vi "RenameDNS.vi"(8 "error in (no error)":errorcluster, 10 "Targets in":T3 {"Filtered Targets"."IP Mode" items=["Static"=1, "DHCP/Link-Local"=2, "Link-Local Only"=4, "DHCP Only"=8]}, 11 "Ctl Refs in":T6) -> (0 "error out":errorcluster, 2 "Targets out":T3 {"Filtered Targets"."IP Mode" items=["Static"=1, "DHCP/Link-Local"=2, "Link-Local Only"=4, "DHCP Only"=8]}, 4 "Buttons out":T2, 5 "Execution State out":T1)   [LabVIEW 2013]
uses:
  Controls/Refs.ctl
  Controls/Button Refs.ctl
  Controls/Tab Ctl Refs.ctl
  types/TabStateType.ctl
  Controls/Indicator Refs.ctl
  Controls/Slider Refs.ctl
  Controls/Control Refs.ctl
  Controls/Targets.ctl
  Controls/Detected.ctl
  types/MAX Sys Cfg Target Information.ctl
  types/ButtonStateType.ctl
  types/ExecutionStateType.ctl
  <vilib>/nisyscfg/Save Changes (System).vi
  <vilib>/nisyscfg/Close (System).vi
  <vilib>/nisyscfg/nisyscfg.lvlib
  <resource>/objmgr/nisysapi.rc
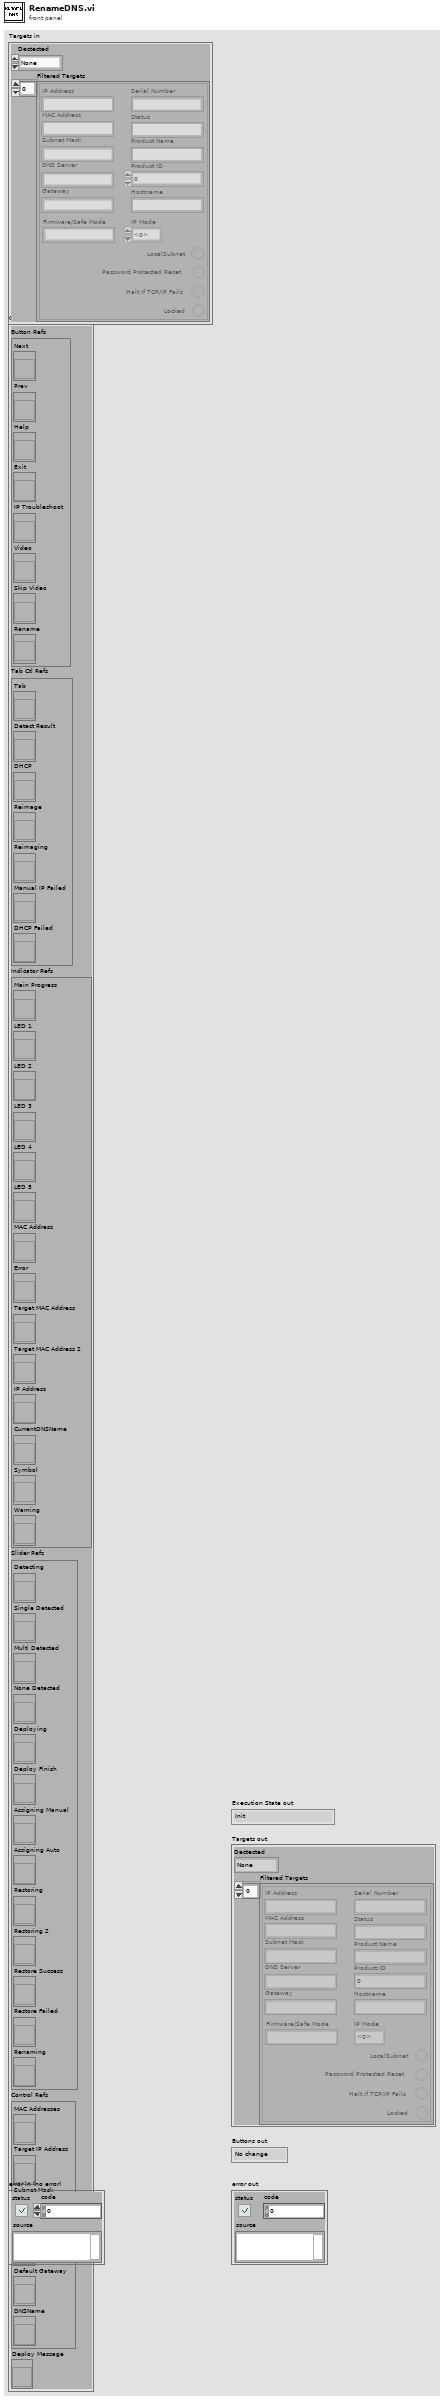
[diagram p1: front panel]
types:
  T1 = typedef "ExecutionStateType.ctl" = enum16{"Init", "Welcome", "Idle", "Detect", "Run Detection", "Detect Fail", "Detect One", "Detect Mult", "Deploy", "DHCP", "Static IP", "Run Deployment", "Connect Verify", "Exit", "Video Wait", "Success", "Troubleshoot", "Troubleshoot 2", "RenameDNS"}
  T2 = typedef "ButtonStateType.ctl" = enum16{"No change", "No Next", "No Prev", "All Disabled", "All Enabled", "Exit Only"}
  T3 = typedef "Targets.ctl" = cluster{"Dectected":T4, "Filtered Targets":T5[]}
  T4 = typedef "Detected.ctl" = enum16{"None", "Failed", "Single", "Multi"}
  T5 = typedef "MAX Sys Cfg Target Information.ctl" = cluster{"MAC Address":string, "IP Address":string, "Status":string, "Product Name":string, "Hostname":string, "Firmware/Safe Mode":string, "Subnet Mask":string, "Gateway":string, "DNS Server":string, "Serial Number":string, "Product ID":u32, "Locked ":bool, "LocalSubnet":bool, "Halt If TCP/IP Fails":bool, "Password Protected Reset":bool, "IP Mode":i32}
  T6 = typedef "Refs.ctl" = cluster{"Button Refs":T7, "Tab Ctl Refs":T8, "Indicator Refs":T9, "Slider Refs":T10, "Control Refs":T11, "Deploy Message":refnum<vi>}
  T7 = typedef "Button Refs.ctl" = cluster{"Next":refnum<vi>, "Prev":refnum<vi>, "Help":refnum<vi>, "Exit":refnum<vi>, "IP Troubleshoot":refnum<vi>, "Video":refnum<vi>, "Skip Video":refnum<vi>, "Rename":refnum<vi>}
  T8 = typedef "Tab Ctl Refs.ctl" = cluster{"Tab":refnum<vi>, "Detect Result":refnum<vi>, "DHCP":refnum<vi>, "Reimage":refnum<vi>, "Reimaging":refnum<vi>, "Manual IP Failed":refnum<vi>, "DHCP Failed":refnum<vi>}
  T9 = typedef "Indicator Refs.ctl" = cluster{"Main Progress":refnum<vi>, "LED 1":refnum<vi>, "LED 2":refnum<vi>, "LED 3":refnum<vi>, "LED 4":refnum<vi>, "LED 5":refnum<vi>, "MAC Address":refnum<vi>, "Error":refnum<vi>, "Target MAC Address":refnum<vi>, "Target MAC Address 2":refnum<vi>, "IP Address":refnum<vi>, "CurrentDNSName":refnum<vi>, "Symbol":refnum<vi>, "Warning":refnum<vi>}
  T10 = typedef "Slider Refs.ctl" = cluster{"Detecting":refnum<vi>, "Single Detected":refnum<vi>, "Multi Detected":refnum<vi>, "None Detected":refnum<vi>, "Deploying":refnum<vi>, "Deploy Finish":refnum<vi>, "Assigning Manual":refnum<vi>, "Assigning Auto":refnum<vi>, "Restoring":refnum<vi>, "Restoring 2":refnum<vi>, "Restore Success":refnum<vi>, "Restore Failed":refnum<vi>, "Renaming":refnum<vi>}
  T11 = typedef "Control Refs.ctl" = cluster{"MAC Addresses":refnum<vi>, "Target IP Address":refnum<vi>, "Subnet Mask":refnum<vi>, "DNS IP":refnum<vi>, "Default Gateway":refnum<vi>, "DNSName":refnum<vi>}
  T12 = typedef "TabStateType.ctl" = enum32{"Welcome", "Instructions", "Detect", "Run Detection", "Detect Result", "Deploy", "Run Deployment", "Connect Verify", "Success", "DHCP", "Troubleshoot", "System Restore", "Error", "Video", "Rename"}
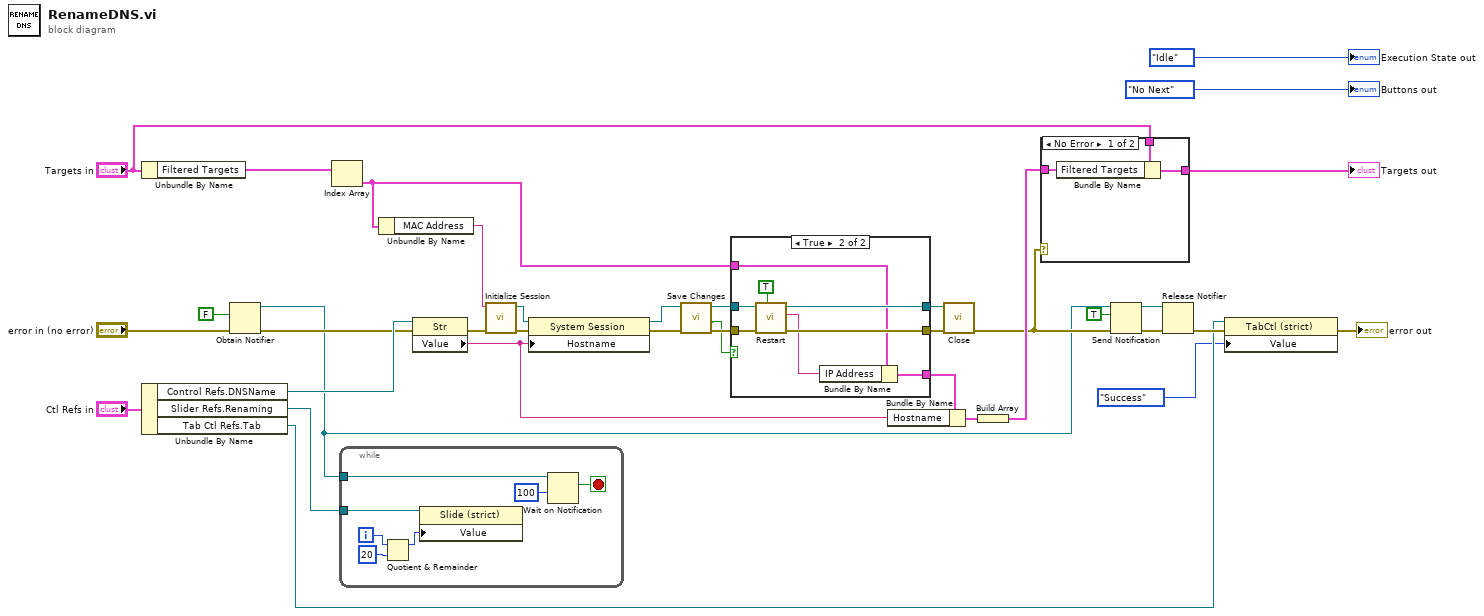
[diagram p0: block diagram]
diagram:
  n1 = Unbundle By Name("Targets in") -> ("Filtered Targets"=w36:T5[])
  n2 = Unbundle By Name("Ctl Refs in") -> ("Control Refs.DNSName"=w22:refnum<vi>, "Slider Refs.Renaming"=w11:refnum<vi>, "Tab Ctl Refs.Tab"=w2:refnum<vi>)
  n3 = Obtain Notifier(notification data type=FALSE ("wait until complete (T)"), error in (no error)="error in (no error)") -> (notifier out=w7:refnum<notifier>, error out=w10:errorcluster)  [unwired: 2 in, 1 out]
  n4 = Index Array(array=w36) -> (element=w25:T5)  [unwired: 1 in]
  n5 = while {
    tunnel: w11 -> [w40]
    tunnel: w7 -> [w39]
    i -> [w42]
    stop <- w37 stop-if-true
    n6 = Quotient & Remainder(x=w42, y=20) -> (x-y*floor(x/y)=w41:i32)  [unwired: 1 out]
    n7 = property class="Slide (strict)"(reference=w40, "Value"=w41) -> ()  [unwired: 1 in, 2 out]
    n8 = Wait on Notification(notifier=w39, timeout in ms (-1)=100) -> (notification=w37:bool)  [unwired: 2 in, 3 out]
  }
  n9 = Unbundle By Name(w25) -> ("MAC Address"=w35:string)
  n10 = property class="Str"(reference=w22, error in=w10) -> (error out=w21:errorcluster, "Value"=w20:string)  [unwired: 1 out]
  n11 = call <vilib>:"Initialize Session.vi"("error in (no error)"=w21, "target (localhost)"=w35) -> ("error out"=w34:errorcluster, "session out"=w33:refnum<k21>)  [unwired: 8 in]
  n12 = property class="System Session"(reference=w33, error in=w34, "Hostname"=w20) -> (reference out=w31:refnum<k21>, error out=w32:errorcluster)
  n13 = call-poly <vilib>:"Save Changes.vi"("error in (no error)"=w32, "session in"=w31) -> ("error out"=w30:errorcluster, "changes require restart"=w29:bool, "session out"=w28:refnum<k21>)  [unwired: 6 in, 1 out]
  n14 = case shown="True" w29 {
    tunnel: w30 -> [w45 w54]
    tunnel: w28 -> [w46 w53]
    tunnel: [w45 w51] -> w27
    tunnel: [w46 w50] -> w26
    tunnel: w25 -> [w44 w49]
    tunnel: [w44 w47] -> w24
    frame False {
    }
    frame True {
      n15 = call <vilib>:"Restart.vi"("wait until complete (T)"=TRUE, "error in (no error)"=w54, "session in"=w53) -> ("error out"=w51:errorcluster, "new IP address"=w48:string, "session out"=w50:refnum<k21>)  [unwired: 6 in]
      n16 = Bundle By Name(cluster=w49, "IP Address"=w48) -> (w47:T5)
    }
  }
  n17 = Bundle By Name(cluster=w24, "Hostname"=w20) -> (w18:T5)
  n18 = call-poly <vilib>:"Close.vi"("error in (no error)"=w27, "session in"=w26) -> ("error out"=w15:errorcluster)  [unwired: 9 in]
  n19 = Build Array(w18) -> (w17:T5[])
  n20 = case shown="No Error" w15 {
    tunnel: "Targets in" -> [w57 w58]
    tunnel: w17 -> [w56 _]
    tunnel: [w55 w58] -> w16
    frame No Error {
      n21 = Bundle By Name(cluster=w57, "Filtered Targets"=w56) -> (w55:T3)
    }
    frame Error {
    }
  }
  "Targets out" <- w16
  n22 = Send Notification(notification=TRUE, notifier=w7, error in (no error)=w15) -> (notifier out=w5:refnum<notifier>, error out=w8:errorcluster)
  n23 = Release Notifier(notifier=w5, error in (no error)=w8) -> (error out=w6:errorcluster)  [unwired: 1 in, 2 out]
  n24 = property class="TabCtl (strict)"(reference=w2, error in=w6, "Value"=TabStateType."Success") -> (error out=→"error out":errorcluster)  [unwired: 1 out]
  "Buttons out" <- ButtonStateType."No Next" ("Buttons out")
  "Execution State out" <- ExecutionStateType."Idle" ("Execution State out")
